vi "Kelvinox_Rotator_Merge_Cluster.vi"(1 "Kelvinox-Rotator-Status":T1={"Angle (deg)"=3.4572, "Target Angle (deg)"=3.4572} {"Target Angle (deg)" format="%4.2g"; "Angle (deg)" format="%4.2g"}, 2 "Kelvinox-Rotator-Control":T2 {"Angle SP" format="%#.2g"}) -> (0 "Kelvinox-Rotator-Cluster":T3={"Angle (deg)"=3.4572, "Target Angle (deg)"=3.4572, "Angle SP"=0.0, "Set Angle SP"=FALSE, "Set Angle to Zero"=FALSE} {"Target Angle (deg)" format="%4.2g"; "Angle SP" format="%#.2g"; "Angle (deg)" format="%4.2g"})   [LabVIEW 2019]
uses:
  Kelvinox/Kelvinox_Rotator_Cluster.ctl
  Kelvinox/Kelvinox_Rotator_Control.ctl
  Kelvinox/Kelvinox_Rotator_Status.ctl
panel:
  # "Kelvinox Rotator"
  # "Kelvinox Rotator"
  # "Kelvinox Rotator"
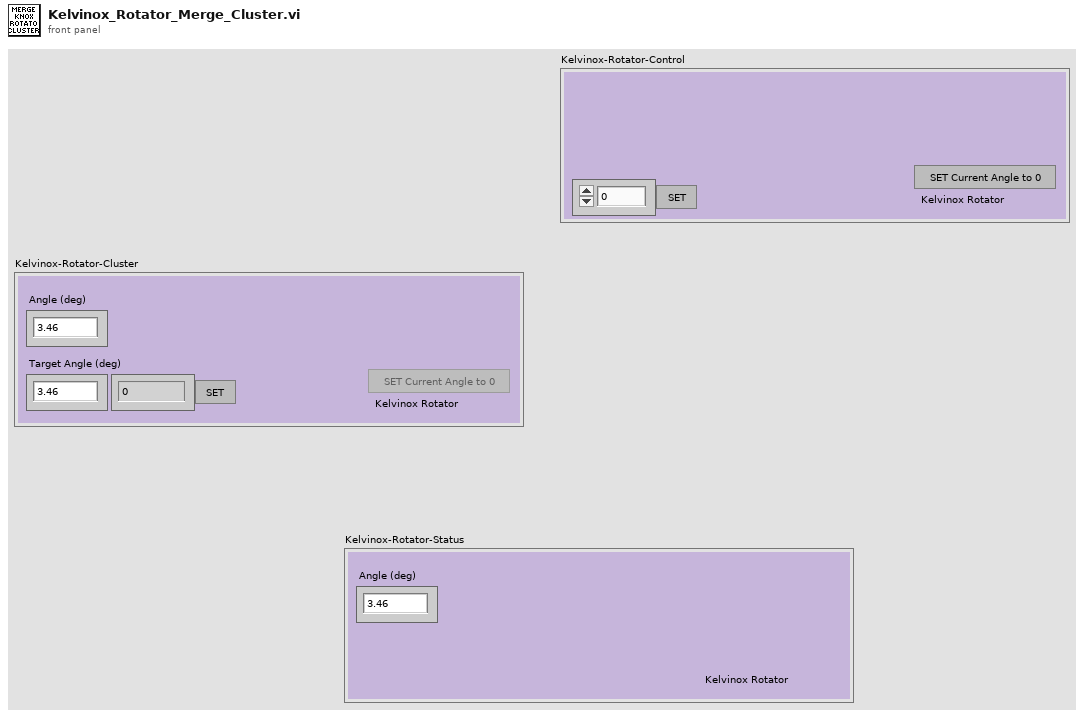
[diagram p1: front panel]
types:
  T1 = typedef "Kelvinox_Rotator_Status.ctl" = cluster{"Angle (deg)":dbl, "Target Angle (deg)":dbl}
  T2 = typedef "Kelvinox_Rotator_Control.ctl" = cluster{"Angle SP":dbl, "Set Angle SP":bool, "Set Angle to Zero":bool}
  T3 = typedef "Kelvinox_Rotator_Cluster.ctl" = cluster{"Angle (deg)":dbl, "Target Angle (deg)":dbl, "Angle SP":dbl, "Set Angle SP":bool, "Set Angle to Zero":bool}
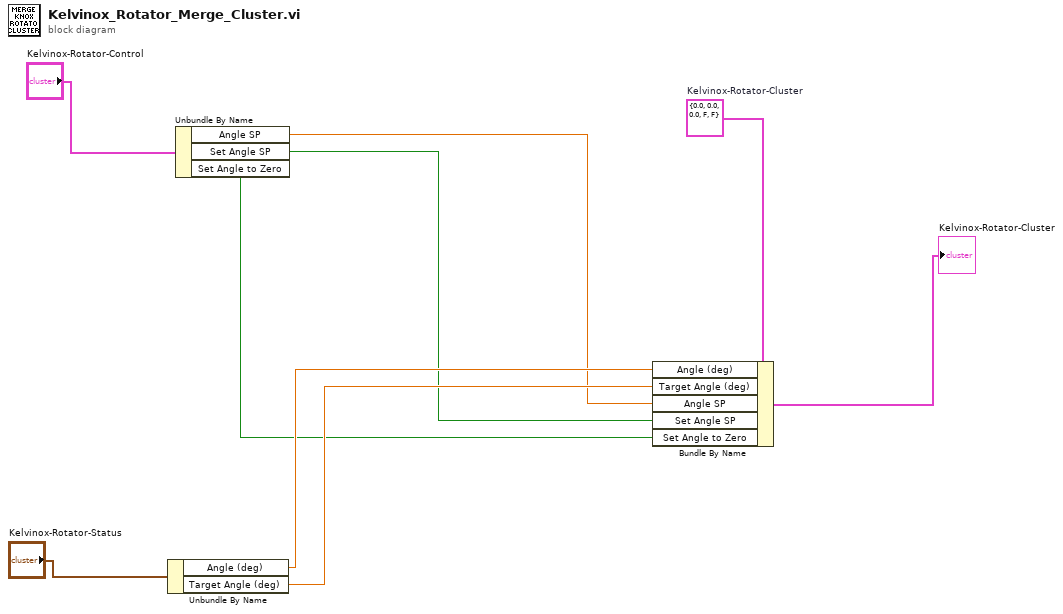
[diagram p0: block diagram]
diagram:
  w7 = T3 {"Angle (deg)"=0.0, "Target Angle (deg)"=0.0, "Angle SP"=0.0, "Set Angle SP"=FALSE, "Set Angle to Zero"=FALSE}  # Kelvinox-Rotator-Cluster
  n1 = Unbundle By Name("Kelvinox-Rotator-Status") -> ("Angle (deg)"=w6:dbl, "Target Angle (deg)"=w5:dbl)
  n2 = Unbundle By Name("Kelvinox-Rotator-Control") -> ("Angle SP"=w4:dbl, "Set Angle SP"=w3:bool, "Set Angle to Zero"=w2:bool)
  n3 = Bundle By Name(cluster=w7, "Angle (deg)"=w6, "Target Angle (deg)"=w5, "Angle SP"=w4, "Set Angle SP"=w3, "Set Angle to Zero"=w2) -> (→"Kelvinox-Rotator-Cluster":T3)
